vi "Measure Supply IV.vi"(0 "Supply Handle in":refnum<k15>, 1 "Channel Name(s)":string, 11 "error in (no error)":errorcluster) -> (4 "Supply Handle out":refnum<k15>, 6 "Measurement Results":T1 {"Power (W)" format="%#_6p"; "Current (A)" format="%#_6p"; "Voltage (V)" format="%#_6p"}, 15 "error out":errorcluster)   [LabVIEW 2019, in "Supply.lvlib"]
uses:
  Supply.lvlib
  Typedefs/Measurement Results.ctl
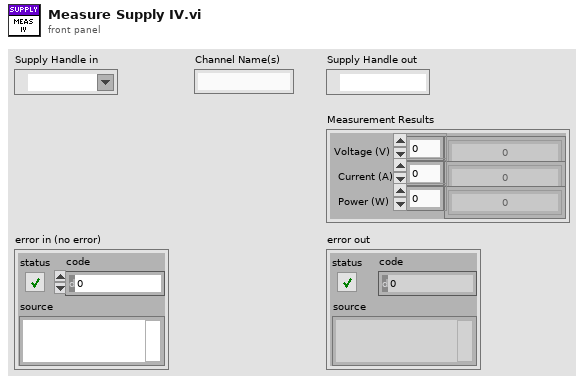
[diagram p1: front panel]
types:
  T1 = typedef "Supply.lvlib/Measurement Results.ctl" = cluster{"Voltage (V)":dbl[], "Current (A)":dbl[], "Power (W)":dbl[]}
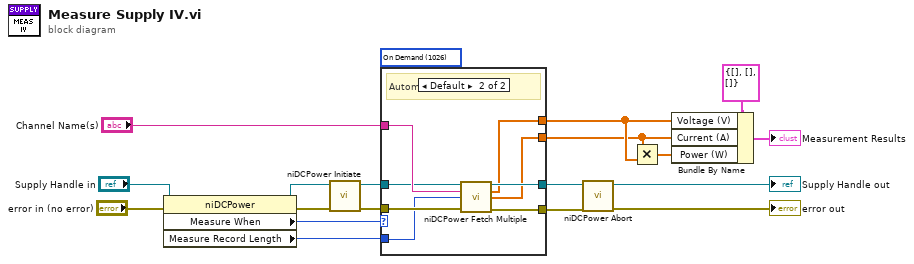
[diagram p0: block diagram]
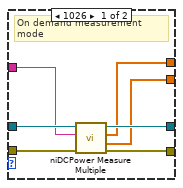
[diagram p2: hidden frame]
diagram:
  (unwired) 1026 items=["Automatically after Source Complete"=1025, "On Demand"=1026, "On Measure Trigger"=1027] ("Measurement:Advanced:Measure When")
  n1 = property class="niDCPower"(reference="Supply Handle in", error in="error in (no error)") -> (reference out=w9:refnum<k15>, error out=w16:errorcluster, "Measure When"=w5:i32, "Measure Record Length"=w1:i32)
  n2 = call <instrlib>:"niDCPower Initiate.vi"("error in (no error)"=w16, "instrument handle"=w9) -> ("error out"=w6:errorcluster, "instrument handle out"=w7:refnum<k15>)  [unwired: 8 in]
  n3 = case shown="Default" w5 {
    tunnel: [w22 w33] -> w17
    tunnel: [w24 w32] -> w15
    tunnel: [w20 w31] -> w4
    tunnel: [w19 w30] -> w2
    tunnel: "Channel Name(s)" -> [w21 w29]
    tunnel: w7 -> [w23 w28]
    tunnel: w6 -> [w25 w27]
    tunnel: w1 -> [_ w26]
    frame 1026 {
      # "On demand measurement mode"
      n4 = call <instrlib>:"niDCPower Measure Multiple.vi"("error in (no error)"=w25, "channel name"=w21, "instrument handle"=w23) -> ("error out"=w24:errorcluster, "current measurements"=w19:dbl[], "voltage measurements"=w20:dbl[], "instrument handle out"=w22:refnum<k15>)  [unwired: 5 in]
    }
    frame Default {
      # "Automatically or Trigger"
      n5 = call <instrlib>:"niDCPower Fetch Multiple.vi"("instrument handle"=w28, "channel name"=w29, "count (1)"=w26, "error in (no error)"=w27) -> ("instrument handle out"=w33:refnum<k15>, "voltage measurements"=w31:dbl[], "current measurements"=w30:dbl[], "error out"=w32:errorcluster)  [unwired: 1 in, 7 out]
    }
  }
  n6 = call <instrlib>:"niDCPower Abort.vi"("error in (no error)"=w15, "instrument handle"=w17) -> ("error out"=→"error out":errorcluster, "instrument handle out"=→"Supply Handle out":refnum<k15>)  [unwired: 8 in]
  n7 = Multiply(x=w2, y=w4) -> (x*y=w3:dbl[])
  n8 = Bundle By Name(cluster=T1 {"Voltage (V)"=[], "Current (A)"=[], "Power (W)"=[]} ("Supply Line Measurements Results"), "Voltage (V)"=w4, "Current (A)"=w2, "Power (W)"=w3) -> (→"Measurement Results":T1)
